vi "通讯类.vi"(8 "error in (no error)":errorcluster caption="错误输入（无错误）", 11 "VISA 输入":refnum<class "VISA.lvclass">) -> (0 "error out":errorcluster caption="错误输出", 3 "VISA 输出":refnum<class "VISA.lvclass">)   [LabVIEW 2016, in "VISA.lvclass"]
uses:
  VISA.lvclass
  <vilib>/Instr/_visa.llb/VISA Configure Serial Port (Instr).vi
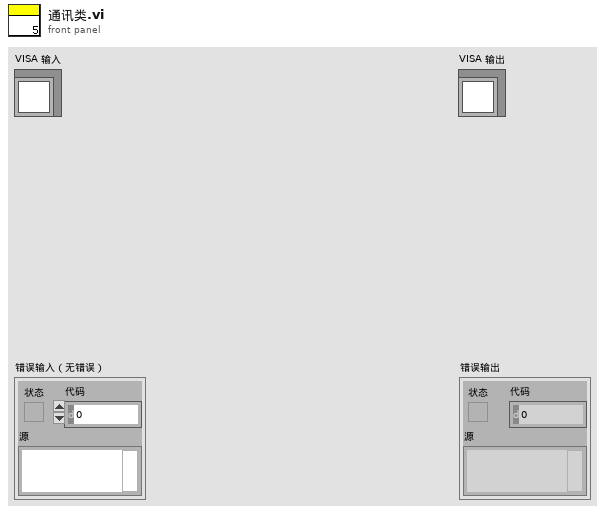
[diagram p1: front panel]
types:
  T1 = cluster{"波特率":u32, "数据比特":u16, "parity (0:none)":u16, "超时":u32}
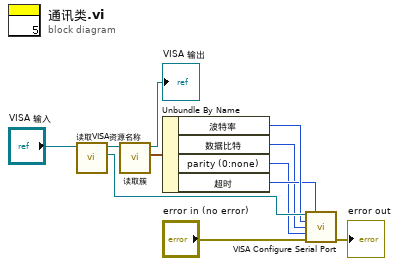
[diagram p0: block diagram]
diagram:
  n1 = call-dynamic "读取VISA资源名称.vi"("VISA输入"="VISA 输入") -> ("VISA资源名称"=w8:refnum<visa-resource-name>, "VISA输出"=w10:refnum<class "VISA.lvclass">)  [unwired: 8 in, 1 out]
  n2 = call-dynamic "读取簇.vi"("VISA输入"=w10) -> ("簇"=w7:T1, "VISA输出"=→"VISA 输出":refnum<class "VISA.lvclass">)  [unwired: 8 in, 1 out]
  n3 = Unbundle By Name(w7) -> ("波特率"=w6:u32, "数据比特"=w4:u16, "parity (0:none)"=w3:u16, "超时"=w5:u32)
  n4 = call-poly "VISA Configure Serial Port"("VISA resource name"=w8, "timeout (10sec)"=w5, "baud rate (9600)"=w6, "data bits (8)"=w4, "parity (0:none)"=w3, "error in (no error)"="error in (no error)") -> ("error out"=→"error out":errorcluster)  [unwired: 8 in, 1 out]
